vi "Read ROM.vi"(7 "1-Wire DIO Pin":refnum<k21>, 8 "error in (no error)":errorcluster) -> (0 "error out":errorcluster, 2 "ROM":u64)   [LabVIEW 2014, in "Maxim 1-Wire.lvlib"]
doc: "READ ROM [33h]\nThis command can only be used when there is one slave on the bus. It allows the bus master to read the slave?s 64-bit ROM code without using the Search ROM procedure. If this command is used when there is more than one slave present on the bus, a data collision will occur when all the slaves attempt to respond at the same time."
uses:
  Maxim 1-Wire.lvlib
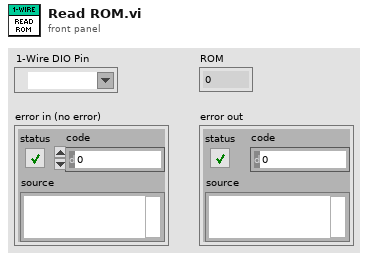
[diagram p1: front panel]
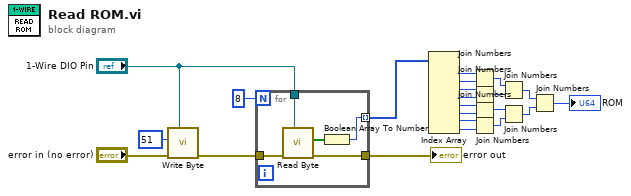
[diagram p0: block diagram]
diagram:
  n1 = call "Write Byte.vi"("1-Wire DIO Pin"="1-Wire DIO Pin", "error in"="error in (no error)", "Tx data"=u8 51 ("Tx data 2")) -> ("error out"=w17:errorcluster)  [unwired: 8 in]
  n2 = for {
    N: 8 -> [_]
    tunnel: w17 -> [w27]
    tunnel: [w26] -> w20
    tunnel: [w24] -> w16 mode=indexing
    tunnel: "1-Wire DIO Pin" -> [w23]
    n3 = call "Read Byte.vi"("1-Wire DIO Pin"=w23, "error in"=w27) -> ("error out"=w26:errorcluster, "Bit Array"=w25:bool[])  [unwired: 8 in]
    n4 = Boolean Array To Number(Boolean array=w25) -> (number=w24:u8)
  }
  "error out" <- w20
  n5 = Index Array(array=w16) -> (element #1=w15:u8, element #2=w14:u8, element #3=w13:u8, element #4=w12:u8, element #5=w11:u8, element #6=w10:u8, element #7=w9:u8, element #8=w8:u8)  [unwired: 8 in]
  n6 = Join Numbers(hi=w15, lo=w14) -> ((hi.lo)=w7:u16)
  n7 = Join Numbers(hi=w13, lo=w12) -> ((hi.lo)=w6:u16)
  n8 = Join Numbers(hi=w11, lo=w10) -> ((hi.lo)=w5:u16)
  n9 = Join Numbers(hi=w9, lo=w8) -> ((hi.lo)=w4:u16)
  n10 = Join Numbers(hi=w7, lo=w6) -> ((hi.lo)=w2:u32)
  n11 = Join Numbers(hi=w5, lo=w4) -> ((hi.lo)=w3:u32)
  n12 = Join Numbers(hi=w2, lo=w3) -> ((hi.lo)=→"ROM":u64)
